vi "compliant arm.vi"(10 "Force Torque":dbl[](array[numeric])) -> ()   [LabVIEW 2010]
panel:
  out "rows 3":dbl
  out "columns":dbl
  out "rows":dbl
  in  "Run":bool
  in  "stop":bool
  out "Position":dbl[][](graph)
  in  "jaw":dbl(knob) scale=0.0..100.0
  in  "elbow":dbl
  in  "slew":dbl
  in  "shoulder":dbl
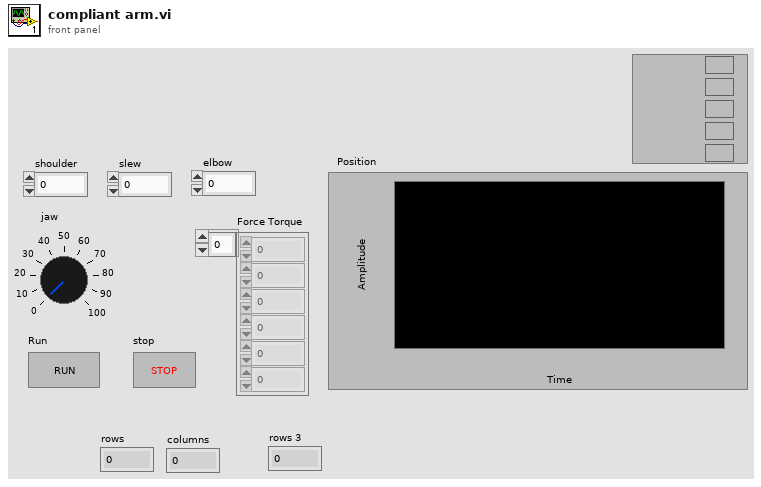
[diagram p1: front panel]
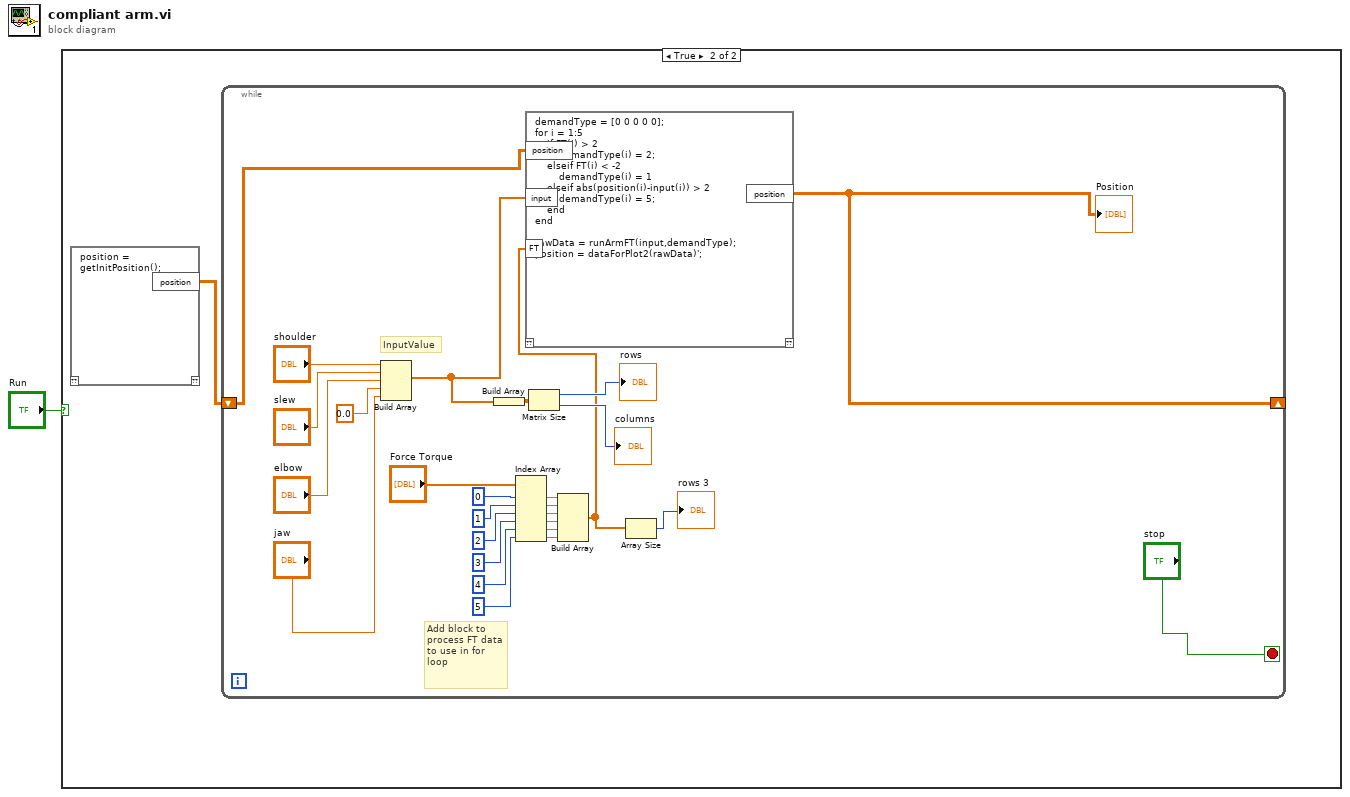
[diagram p0: block diagram]
diagram:
  n1 = case shown="True" "Run" {
    frame False {
    }
    frame True {
      n2 = script code="position = getInitPosition();"() -> ("position"=w2:dbl[][])  [unwired: 1 in, 1 out]
      n3 = while {
        shift-right: [w3] -> _
        shift-left: w2 -> [w4]
        stop <- "stop" stop-if-true
        # "Add block to process FT data to use in for loop"
        # "InputValue"
        n4 = Build Array("shoulder", "slew", "elbow", 0.0 ("element"), "jaw") -> (w20:dbl[])
        n5 = Build Array(w20) -> (w24:dbl[][])
        n6 = Index Array(array="Force Torque", index #1=0 ("index"), index #2=1 ("index"), index #3=2 ("index"), index #4=3 ("index"), index #5=4 ("index"), index #6=5 ("index")) -> (element #1=w17:dbl, element #2=w16:dbl, element #3=w15:dbl, element #4=w14:dbl, element #5=w13:dbl, element #6=w12:dbl)
        n7 = Matrix Size(0:w24) -> (1:→"rows":i32, 2:→"columns":i32)
        n8 = Build Array(w17, w16, w15, w14, w13, w12) -> (w5:dbl[])
        n9 = script code="demandType = [0 0 0 0 0];\nfor i = 1:5\n    if FT(i) > 2\n        demandType(i) = 2;\n    elseif FT(i) < -2\n        demandType(i) = 1\n    elseif abs(position(i)-input(i)) > 2\n        demandType(i) = 5;\n    end\nend\n\nrawData = runArmFT(input,demandType);\nposition = dataForPlot2(rawData)';"("position"=w4, "input"=w20, "FT"=w5) -> ("position"=w3:dbl[][])  [unwired: 1 in, 1 out]
        "Position" <- w3
        n10 = Array Size(array=w5) -> (size(s)=→"rows 3":i32)
      }
    }
  }
